vi "Get Project Targets.vi"(8 "error in":errorcluster, 11 "Project in":refnum<vi>) -> (0 "error out":errorcluster, 3 "Targets":string[](array[string]))   [LabVIEW 2020, in "Panther Dashboard.lvlib"]
uses:
  Panther Dashboard.lvlib
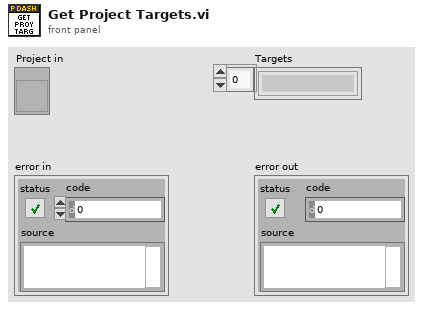
[diagram p1: front panel]
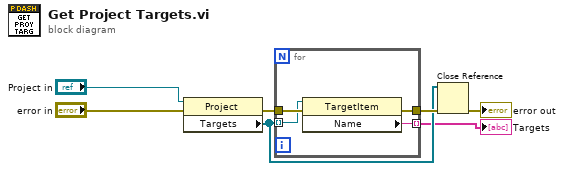
[diagram p0: block diagram]
diagram:
  n1 = property class="Project"(reference="Project in", error in="error in") -> (error out=w4:errorcluster, "Targets"=w3:refnum<vi>[])  [unwired: 1 out]
  n2 = for {
    tunnel: w3 -> [w9] mode=indexing
    tunnel: [w8] -> w2 mode=indexing
    tunnel: w4 -> [w11]
    tunnel: [w10] -> w7
    n3 = property class="TargetItem"(reference=w9, error in=w11) -> (error out=w10:errorcluster, "Name"=w8:string)  [unwired: 1 out]
  }
  "Targets" <- w2
  n4 = Close Reference(reference=w3, error in (no error)=w7) -> (error out=→"error out":errorcluster)
